vi "projet V11.vi"() -> ()   [LabVIEW 2020]
uses:
  <vilib>/MakerHub/LINX/Public/Peripherals/Analog/Analog Read 1 Chan.vi
  <vilib>/MakerHub/LINX/Public/Peripherals/Analog/Analog Read N Chans.vi
  <vilib>/MakerHub/LINX/Private/Local IO/LinxAnalogRead.vi
  <vilib>/MakerHub/LINX/Public/Utilities/Check Channel.vi
  <vilib>/MakerHub/LINX/Public/Utilities/Open Serial.vi
  <vilib>/MakerHub/LINX/Private/Utilties/Generate Error.vi
  <vilib>/ptbypt/NI_PtbyPt.lvlib
  <vilib>/MakerHub/LINX/LMH-LINX.lvlib
panel:
  out "Loop Rate (Hz)":u32
  in  "Serial Port 2":refnum<visa-resource-name>
  out "Voltage":dbl
  out "mean":dbl caption="moyenne accéléromètre" format="%0.2f"
  out "Pas de Y":dbl
  out "SCORE":dbl
  out "Y":dbl
  in  "Niveau de difficulté":dbl(knob) scale=200.0..100.0
  out "X":dbl
  out "?":dbl(slide) scale=0.0..5.0
  out "?":cluster{dbl[], dbl[]}(graph)
  out "?":string
  # "Attention: veuillez choisir un niveau de difficulté avant de commencer"
  # "coordonées de la balle"
  # "Connexion à l'accéléromètre"
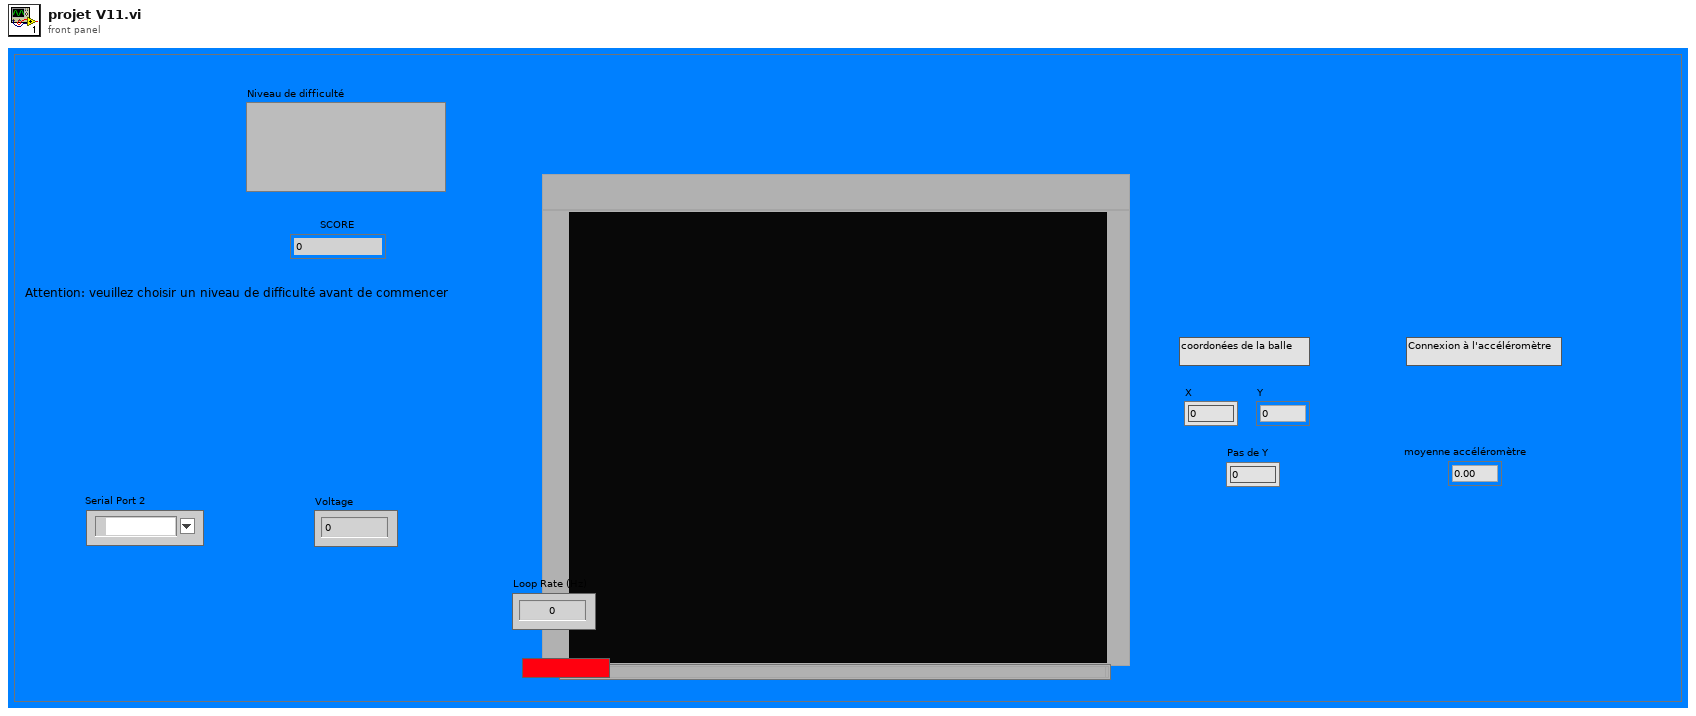
[diagram p1: front panel]
types:
  T1 = typedef "LMH-LINX.lvlib/LINX Ref.ctl" = cluster{"IO":T2, "Interface":T3, "LINX Device Config":T4}
  T2 = typedef "LMH-LINX.lvlib/Platform.ctl" = enum16{"Remote", "Local"}
  T3 = typedef "LMH-LINX.lvlib/Interface.ctl" = enum16{"Serial", "TCP"}
  T4 = typedef "LMH-LINX.lvlib/Device.lvlib/LINX Device Config.ctl" = cluster{"Interface":T3, "COM Port":refnum<visa-resource-name>, "TCP Configuration":T5, "Device Family":u8, "Device ID":u8, "Device Name":string, "TCP Ref":refnum<k5>, "Channels":T6}
  T5 = typedef "LMH-LINX.lvlib/Device.lvlib/TCP Config.ctl" = cluster{"IP Address":string, "Port":u16}
  T6 = typedef "LMH-LINX.lvlib/Channels.ctl" = cluster{"DI":u8[], "DO":u8[], "AI":u8[], "AO":u8[], "PWM":u8[], "QE":u8[], "UART":u8[], "I2C 2":u8[], "SPI":u8[], "CAN":u8[], "Servo":u8[], "AI Ref (V)":dbl, "AI Resolution (Bits)":u8, "AO Ref (V)":dbl, "AO Resolution (Bits)":u8}
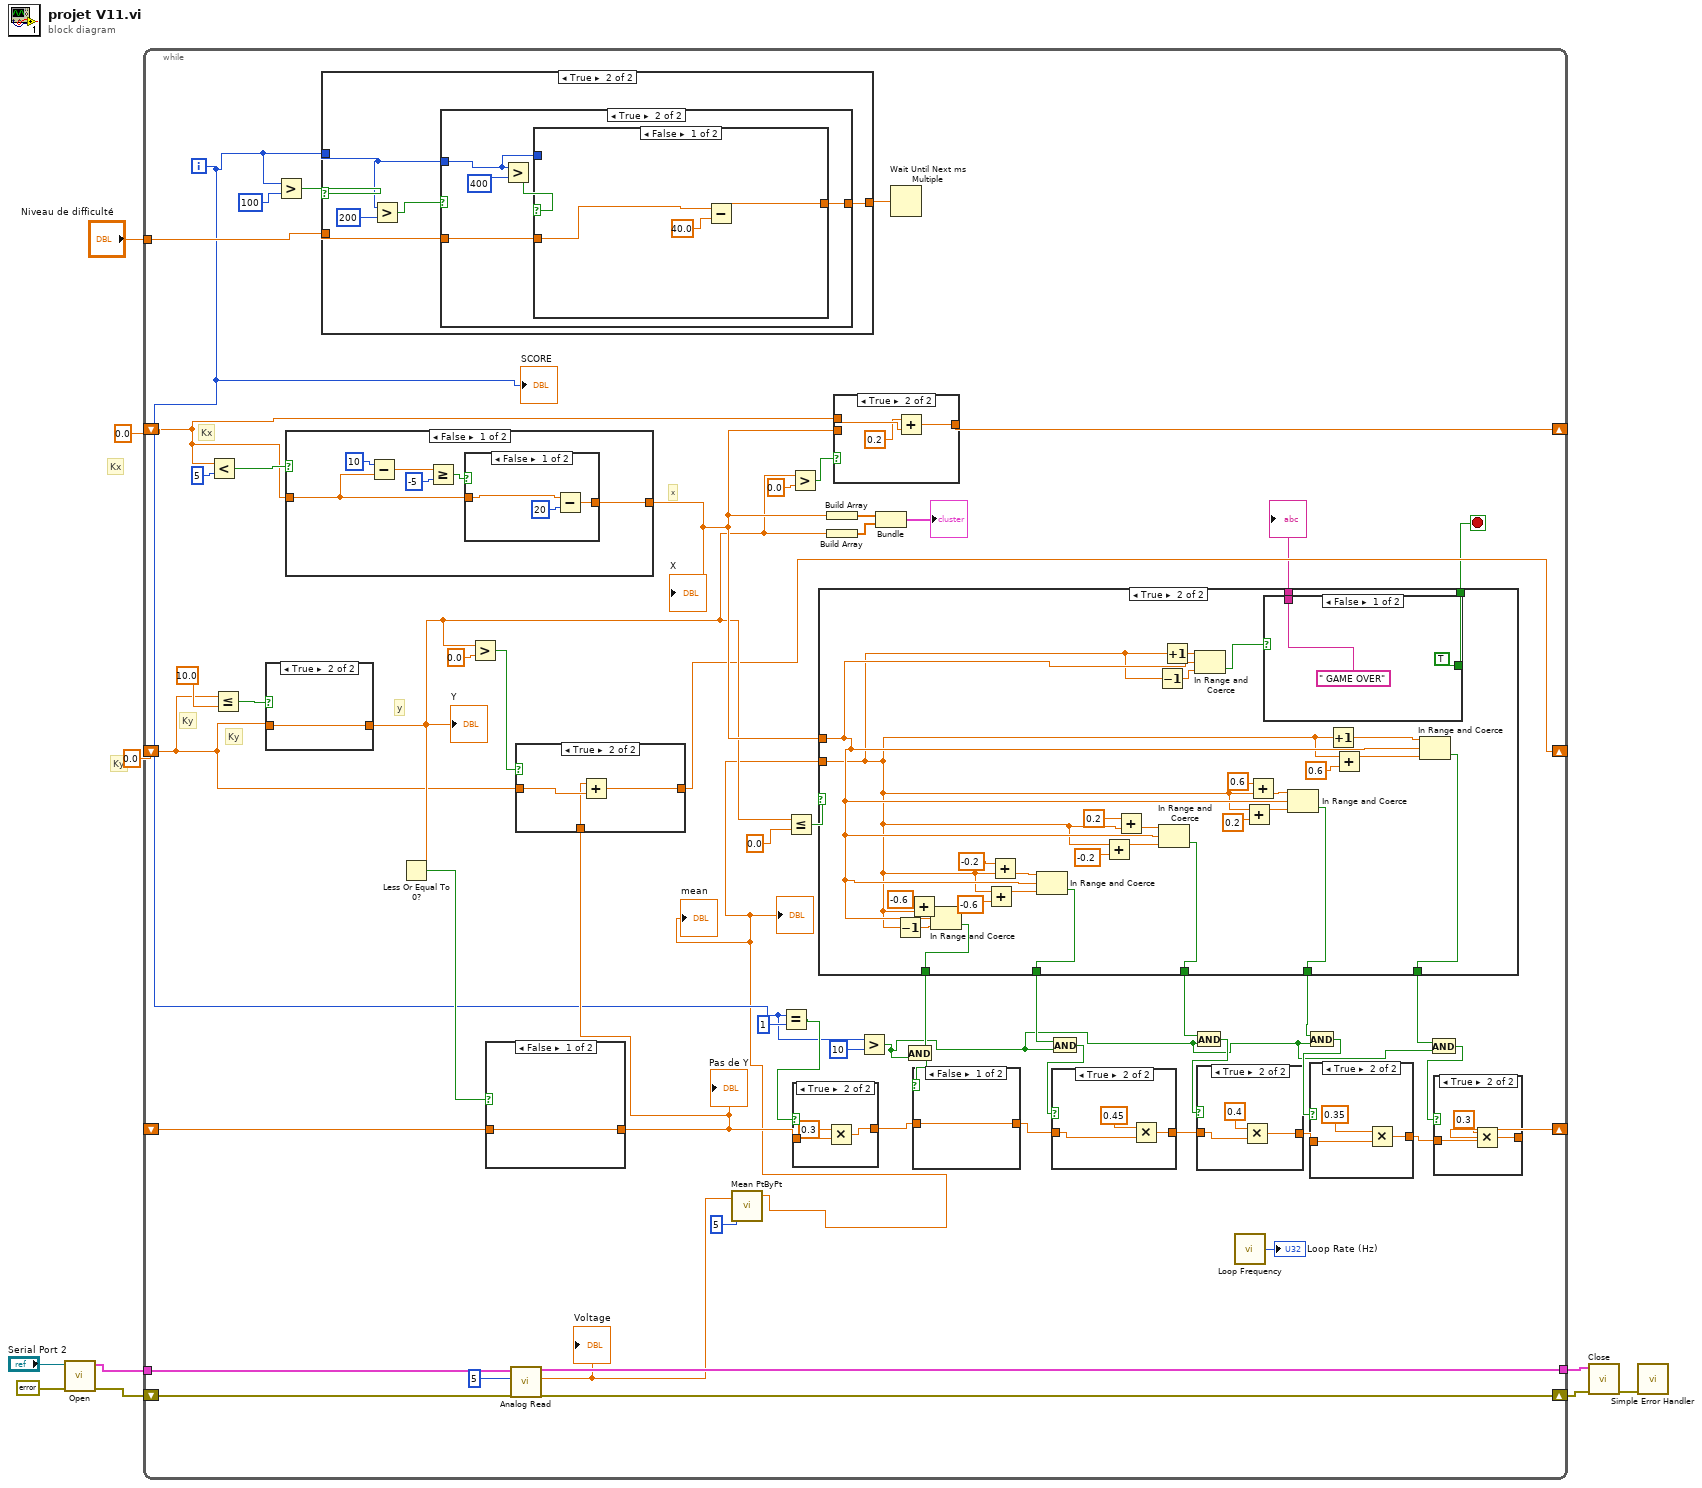
[diagram p0: block diagram]
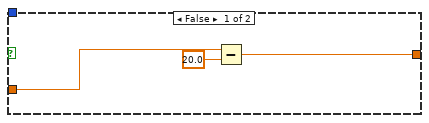
[diagram p6: hidden frame]
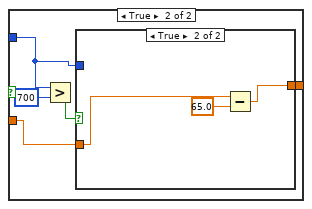
[diagram p7: hidden frame]
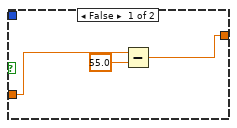
[diagram p8: hidden frame]
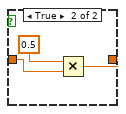
[diagram p11: hidden frame]
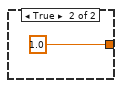
[diagram p12: hidden frame]
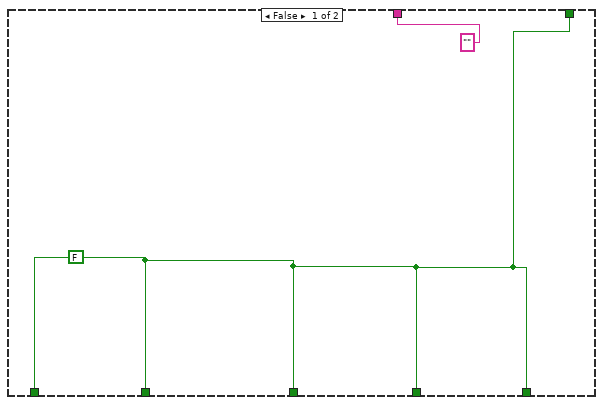
[diagram p13: hidden frame]
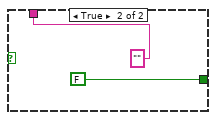
[diagram p14: hidden frame]
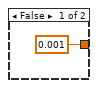
[diagram p15: hidden frame]
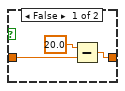
[diagram p17: hidden frame]
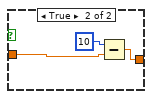
[diagram p18: hidden frame]
diagram:
  # "Kx"
  # "Ky"
  n1 = call-poly <vilib>:"Open.vi"("Error In"=errorcluster {"status"=FALSE, "code"=0, "source"=""}, "Serial Port"="Serial Port 2") -> ("Error Out"=w4:errorcluster, "LINX Resource"=w5:T1)  [unwired: 7 in, 1 out]
  n2 = while {
    shift-right: [w57] -> _
    shift-left: 0.0 -> [w25]
    shift-right: [w21] -> _
    shift-left: 0.0 -> [w52]
    shift-right: [w42] -> _
    shift-left: _ -> [w55]
    tunnel: "Niveau de difficulté" -> [w46]
    tunnel: w5 -> [w16]
    tunnel: [w14] -> w2
    shift-right: [w12] -> w1
    shift-left: w4 -> [w15]
    i -> [w24]
    stop <- w20 stop-if-true
    # "Kx"
    # "x"
    # "Ky"
    # "y"
    # "Ky"
    n3 = Less?(x=w25, y=5) -> (x < y?=w68:bool)
    n4 = Less Or Equal?(x=w52, y=10.0) -> (x <= y?=w66:bool)
    n5 = case shown="True" w66 {
      tunnel: w52 -> [w168 w170]
      tunnel: [w169 w170] -> w53
      frame False {
        n6 = Subtract(x=20.0, y=w168) -> (x-y=w169:dbl)
      }
      frame True {
      }
    }
    "Y" <- w53
    n7 = Greater?(x=w24, y=100) -> (0:w44:bool)
    n8 = case shown="False" w68 {
      tunnel: w25 -> [w175 w183]
      tunnel: [w176 w183] -> w56
      frame False {
        n9 = Subtract(x=10, y=w175) -> (x-y=w172:dbl)
        n10 = Greater Or Equal?(x=w172, y=-5) -> (x >= y?=w173:bool)
        n11 = case shown="False" w173 {
          tunnel: [w179 w182] -> w176
          tunnel: w175 -> [w178 w181]
          frame False {
            n12 = Subtract(x=w178, y=20) -> (x-y=w179:dbl)
          }
          frame True {
            n13 = Subtract(x=10, y=w181) -> (x-y=w182:dbl)
          }
        }
      }
      frame True {
      }
    }
    "X" <- w56
    n14 = case shown="True" w44 {
      tunnel: w46 -> [w81 w85]
      tunnel: [w81 w83] -> w43
      tunnel: w24 -> [_ w82]
      frame False {
      }
      frame True {
        n15 = Greater?(x=w82, y=200) -> (0:w84:bool)
        n16 = case shown="True" w84 {
          tunnel: w85 -> [w89 w92]
          tunnel: [w88 w91] -> w83
          tunnel: w82 -> [_ w90]
          frame False {
            n17 = Subtract(x=w89, y=20.0) -> (x-y=w88:dbl)
          }
          frame True {
            n18 = Greater?(x=w90, y=400) -> (0:w93:bool)
            n19 = case shown="False" w93 {
              tunnel: w92 -> [w96 w101]
              tunnel: [w97 w98] -> w91
              tunnel: w90 -> [_ w100]
              frame False {
                n20 = Subtract(x=w96, y=40.0) -> (x-y=w97:dbl)
              }
              frame True {
                n21 = Greater?(x=w100, y=700) -> (0:w99:bool)
                n22 = case shown="True" w99 {
                  tunnel: w101 -> [w105 w108]
                  tunnel: w100 -> [_ _]
                  tunnel: [w104 w107] -> w98
                  frame False {
                    n23 = Subtract(x=w105, y=55.0) -> (x-y=w104:dbl)
                  }
                  frame True {
                    n24 = Subtract(x=w108, y=65.0) -> (x-y=w107:dbl)
                  }
                }
              }
            }
          }
        }
      }
    }
    n25 = Less Or Equal To 0?(x=w53) -> (x <= 0?=w54:bool)
    n26 = Greater?(x=w53, y=0.0) -> (0:w61:bool)
    n27 = case shown="False" w54 {
      tunnel: [w121 1.0] -> w49
      tunnel: w55 -> [w121 _]
      frame False {
      }
      frame True {
      }
    }
    "Pas de Y" <- w49
    n28 = call-poly <vilib>:"Analog Read.vi"("Error In"=w15, "Analog Channel"=u8 5, "LINX Resource"=w16) -> ("Error Out"=w12:errorcluster, "Voltage"=w11:dbl, "LINX Resource"=w14:T1)  [unwired: 5 in, 1 out]
    "Voltage" <- w11
    n29 = case shown="True" w61 {
      tunnel: w52 -> [_ w162]
      tunnel: [0.001 w161] -> w21
      tunnel: w49 -> [_ w160]
      frame False {
      }
      frame True {
        n30 = Add(x=w160, y=w162) -> (x+y=w161:dbl)
      }
    }
    n31 = call <vilib>:"Mean PtByPt.vi"("x"=w11, "sample length"=5) -> ("mean"=w18:dbl)  [unwired: 2 in, 1 out]
    "?" <- w18
    "mean" <- w18
    n32 = Equal?(x=w24, y=1) -> (x = y?=w48:bool)
    n33 = Less Or Equal?(x=w53, y=0.0) -> (x <= y?=w23:bool)
    n34 = Greater?(x=w53, y=0.0) -> (0:w63:bool)
    n35 = case shown="True" w48 {
      tunnel: [w109 w111] -> w50
      tunnel: w49 -> [w109 w112]
      frame False {
      }
      frame True {
        n36 = Multiply(x=0.3, y=w112) -> (x*y=w111:dbl)
      }
    }
    n37 = case shown="True" w23 {
      tunnel: w18 -> [_ w127]
      tunnel: w56 -> [_ w128]
      tunnel: [w124 w154] -> w36
      tunnel: [w124 w135] -> w34
      tunnel: [w124 w132] -> w28
      tunnel: [w124 w133] -> w29
      tunnel: [w124 w134] -> w32
      tunnel: [w124 w126] -> w20
      tunnel: ["" w125] -> w19
      frame False {
        w124 = FALSE
      }
      frame True {
        n38 = Decrement(x=w127) -> (x-1=w136:dbl)
        n39 = Add(x=-0.6, y=w127) -> (x+y=w138:dbl)
        n40 = In Range and Coerce(upper limit=w138, x=w128, lower limit=w136) -> (In Range?=w154:bool)  [unwired: 1 out]
        n41 = Add(x=w127, y=-0.6) -> (x+y=w140:dbl)
        n42 = Add(x=-0.2, y=w127) -> (x+y=w142:dbl)
        n43 = In Range and Coerce(upper limit=w142, x=w128, lower limit=w140) -> (In Range?=w135:bool)  [unwired: 1 out]
        n44 = Add(x=w127, y=-0.2) -> (x+y=w144:dbl)
        n45 = Add(x=0.2, y=w127) -> (x+y=w146:dbl)
        n46 = Decrement(x=w127) -> (x-1=w130:dbl)
        n47 = In Range and Coerce(upper limit=w146, x=w128, lower limit=w144) -> (In Range?=w134:bool)  [unwired: 1 out]
        n48 = Increment(x=w127) -> (x+1=w131:dbl)
        n49 = In Range and Coerce(upper limit=w131, x=w128, lower limit=w130) -> (In Range?=w129:bool)  [unwired: 1 out]
        n50 = Add(x=w127, y=0.2) -> (x+y=w149:dbl)
        n51 = Add(x=0.6, y=w127) -> (x+y=w150:dbl)
        n52 = case shown="False" w129 {
          tunnel: [TRUE FALSE] -> w126
          tunnel: [" GAME OVER" ""] -> w125
          frame False {
          }
          frame True {
          }
        }
        n53 = In Range and Coerce(upper limit=w150, x=w128, lower limit=w149) -> (In Range?=w133:bool)  [unwired: 1 out]
        n54 = Increment(x=w127) -> (x+1=w153:dbl)
        n55 = Add(x=w127, y=0.6) -> (x+y=w152:dbl)
        n56 = In Range and Coerce(upper limit=w153, x=w128, lower limit=w152) -> (In Range?=w132:bool)  [unwired: 1 out]
      }
    }
    "?" <- w19
    n57 = Build Array(w56) -> (w58:dbl[])
    n58 = Build Array(w53) -> (w59:dbl[])
    n59 = case shown="True" w63 {
      tunnel: w25 -> [_ w166]
      tunnel: [w163 w165] -> w57
      tunnel: w56 -> [w163 _]
      frame False {
      }
      frame True {
        n60 = Add(x=0.2, y=w166) -> (x+y=w165:dbl)
      }
    }
    n61 = Greater?(x=w24, y=10) -> (0:w26:bool)
    n62 = Bundle(w58, w59) -> (→"?":cluster{dbl[], dbl[]})  [unwired: 1 in]
    n63 = Wait Until Next ms Multiple(millisecond multiple=w43) -> ()  [unwired: 1 out]
    n64 = And(x=w36, y=w26) -> (x .and. y?=w35:bool)
    n65 = case shown="False" w35 {
      tunnel: w50 -> [w117 w120]
      tunnel: [w117 w119] -> w41
      frame False {
      }
      frame True {
        n66 = Multiply(x=0.5, y=w120) -> (x*y=w119:dbl)
      }
    }
    n67 = And(x=w34, y=w26) -> (x .and. y?=w33:bool)
    n68 = case shown="True" w33 {
      tunnel: w41 -> [w77 w79]
      tunnel: [w77 w78] -> w40
      frame False {
      }
      frame True {
        n69 = Multiply(x=0.45, y=w79) -> (x*y=w78:dbl)
      }
    }
    n70 = And(x=w32, y=w26) -> (x .and. y?=w31:bool)
    n71 = case shown="True" w31 {
      tunnel: w40 -> [w73 w74]
      tunnel: [w73 w75] -> w39
      frame False {
      }
      frame True {
        n72 = Multiply(x=0.4, y=w74) -> (x*y=w75:dbl)
      }
    }
    n73 = call <vilib>:"Loop Frequency.vi"() -> ("Loop Rate (Hz)"=→"Loop Rate (Hz)":u32)
    n74 = And(x=w29, y=w26) -> (x .and. y?=w30:bool)
    n75 = case shown="True" w30 {
      tunnel: w39 -> [w69 w71]
      tunnel: [w69 w70] -> w38
      frame False {
      }
      frame True {
        n76 = Multiply(x=0.35, y=w71) -> (x*y=w70:dbl)
      }
    }
    n77 = And(x=w28, y=w26) -> (x .and. y?=w27:bool)
    n78 = case shown="True" w27 {
      tunnel: [w113 w116] -> w42
      tunnel: w38 -> [w113 w114]
      frame False {
      }
      frame True {
        n79 = Multiply(x=0.3, y=w114) -> (x*y=w116:dbl)
      }
    }
    "SCORE" <- w24
  }
  n80 = call <vilib>:"Close.vi"("Error In"=w1, "LINX Resource"=w2) -> ("Error Out"=w3:errorcluster)  [unwired: 9 in]
  n81 = call <vilib>:"Simple Error Handler.vi"("error in (no error)"=w3) -> ()  [unwired: 4 in, 5 out]
